vi "File IO.vi"(8 "error in":errorcluster, 9 "This Scan #":u32, 11 "File IO in":refnum<class "File IO.lvclass">) -> (0 "error out":errorcluster, 3 "File IO out":refnum<class "File IO.lvclass">)   [LabVIEW 2009, in "File IO.lvclass"]
uses:
  File IO.lvclass
  File IO.lvclass/File IO.ctl
  Global/File Locations.vi
panel:
  out "Temp File Path":path
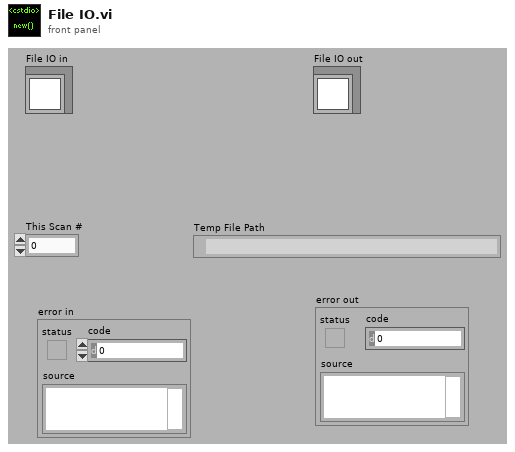
[diagram p1: front panel]
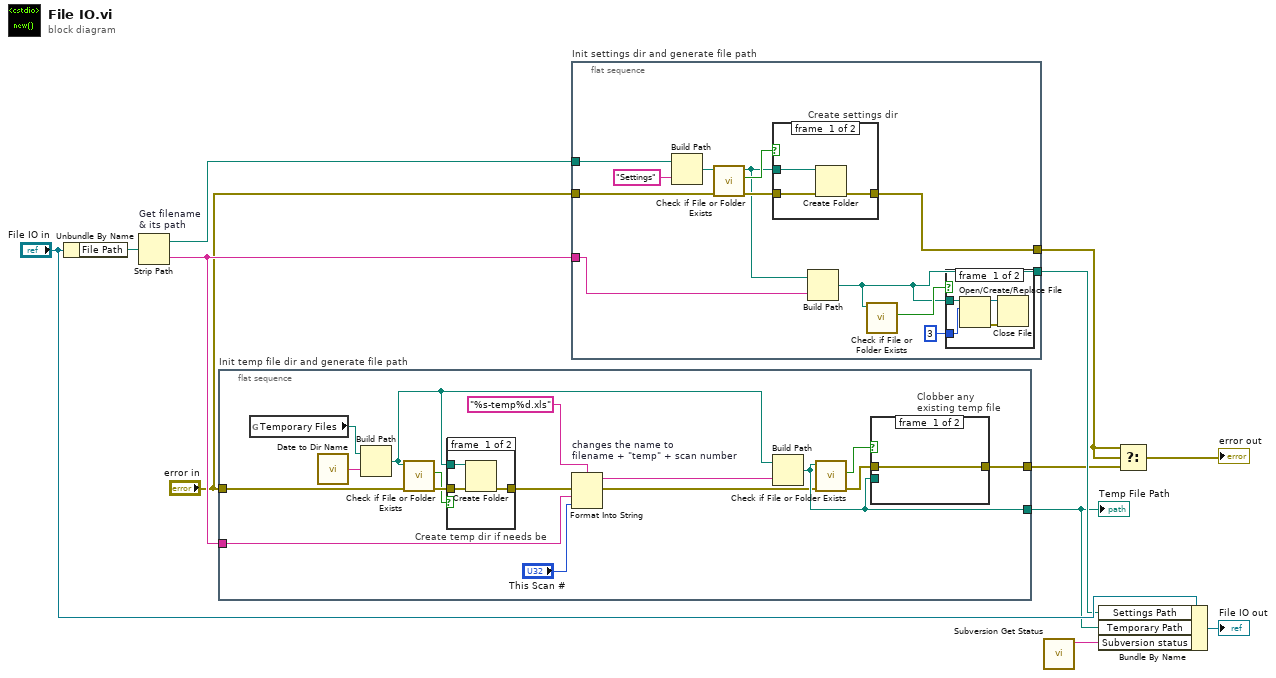
[diagram p0: block diagram]
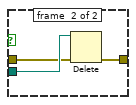
[diagram p3: hidden frame]
diagram:
  n1 = Unbundle By Name("File IO in") -> ("File Path"=w12:path)
  n2 = Strip Path "Get filename\n& its path"(path=w12) -> (stripped path=w9:path, name=w8:string)
  n3 = flat-sequence "Init temp file dir and generate file path" {
    tunnel: [w22] -> w5
    tunnel: [w21] -> w4
    tunnel: w8 -> [w16]
    tunnel: "error in" -> [w13]
    frame #0 {
      n4 = global read "File Locations.vi" "Temporary Files"() -> (w26:path)
      n5 = call "Date to Dir Name.vi"() -> ("Dir Name"=w25:string)
      n6 = Build Path(base path=w26, name or relative path=w25) -> (appended path=w17:path)
      n7 = call <vilib>:"Check if File or Folder Exists.vi"("error in (no error)"=w13, "path"=w17) -> ("error out"=w20:errorcluster, "file or folder exists?"=w18:bool)  [unwired: 8 out]
      n8 = case "Create temp dir if needs be" shown="False" w18 {
        tunnel: w20 -> [w31 w32]
        tunnel: w17 -> [w30 _]
        tunnel: [w29 w32] -> w15
        frame #0 {
          n9 = Create Folder(path (use dialog)=w30, error in=w31) -> (error out=w29:errorcluster)  [unwired: 3 out]
        }
        frame #1 {
        }
      }
      n10 = Format Into String "changes the name to \nfilename + \"temp\" + scan number"(format string="%s-temp%d.xls", error in=w15, w16, "This Scan #") -> (resulting string=w24:string, error out=w14:errorcluster)  [unwired: 1 in]
      n11 = Build Path(base path=w17, name or relative path=w24) -> (appended path=w22:path)
      n12 = call <vilib>:"Check if File or Folder Exists.vi"("error in (no error)"=w14, "path"=w22) -> ("error out"=w19:errorcluster, "file or folder exists?"=w23:bool)  [unwired: 8 out]
      n13 = case "Clobber any\nexisting temp file" shown="True" w23 {
        tunnel: w22 -> [_ w36]
        tunnel: w19 -> [w33 w35]
        tunnel: [w33 w34] -> w21
        frame #0 {
        }
        frame #1 {
          n14 = Delete(path (use dialog)=w36, error in=w35) -> (error out=w34:errorcluster)  [unwired: 5 out]
        }
      }
    }
  }
  n15 = flat-sequence "Init settings dir and generate file path" {
    tunnel: w9 -> [w48]
    tunnel: w8 -> [w40]
    tunnel: [w38] -> w7
    tunnel: "error in" -> [w42]
    tunnel: [w41] -> w3
    frame #0 {
      n16 = Build Path(base path=w48, name or relative path="Settings") -> (appended path=w46:path)
      n17 = call <vilib>:"Check if File or Folder Exists.vi"("error in (no error)"=w42, "path"=w46) -> ("error out"=w44:errorcluster, "file or folder exists?"=w45:bool, "dup path"=w43:path)  [unwired: 7 out]
      n18 = case "Create settings dir" shown="False" w45 {
        tunnel: w44 -> [w55 w56]
        tunnel: [w54 w56] -> w41
        tunnel: w43 -> [w53 _]
        frame #0 {
          n19 = Create Folder(path (use dialog)=w53, error in=w55) -> (error out=w54:errorcluster)  [unwired: 3 out]
        }
        frame #1 {
        }
      }
      n20 = Build Path(base path=w43, name or relative path=w40) -> (appended path=w38:path)
      n21 = call <vilib>:"Check if File or Folder Exists.vi"("path"=w38) -> ("file or folder exists?"=w39:bool)  [unwired: 8 in, 2 out]
      n22 = case shown="False" w39 {
        tunnel: w38 -> [w52 _]
        tunnel: 3 -> [w51 _]
        frame #0 {
          n23 = Open/Create/Replace File(file path (use dialog)=w52, operation (0:open)=w51) -> (refnum out=w49:refnum<file>, error out=w50:errorcluster)  [unwired: 4 in, 1 out]
          n24 = Close File(refnum=w49, error in=w50) -> ()  [unwired: 2 out]
        }
        frame #1 {
        }
      }
    }
  }
  n25 = call "Subversion Get Status.vi"() -> ("SVN Status"=w1:string)  [unwired: 11 out]
  n26 = Bundle By Name(cluster="File IO in", "Settings Path"=w7, "Temporary Path"=w5, "Subversion status"=w1) -> (→"File IO out":refnum<class "File IO.lvclass">)
  n27 = Select(t=w3, s=w3, f=w4) -> (s? t:f=→"error out":errorcluster)
  "Temp File Path" <- w5
